vi "QWTB Algorithms Filter Set Config.vi"(9 "new algorithm config section data":string, 10 "algorithm name":string, 11 "info data":string) -> (3 "info data out":string)   [LabVIEW 2020]
uses:
  octave/infolib/infolib.lvlib
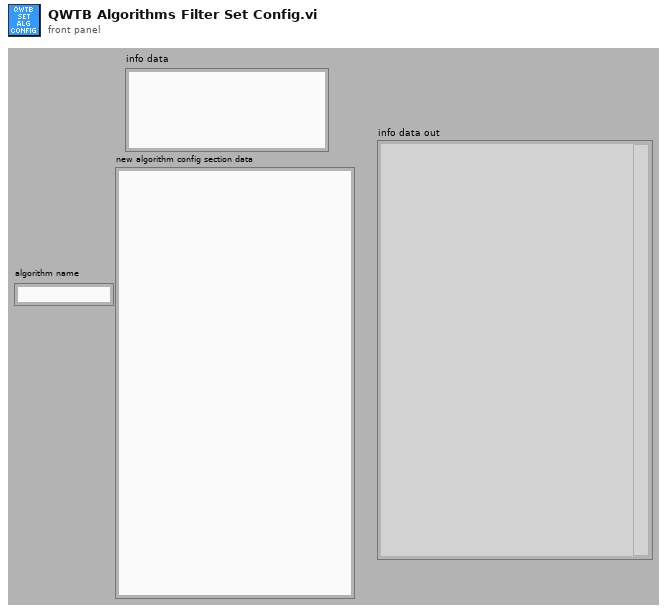
[diagram p1: front panel]
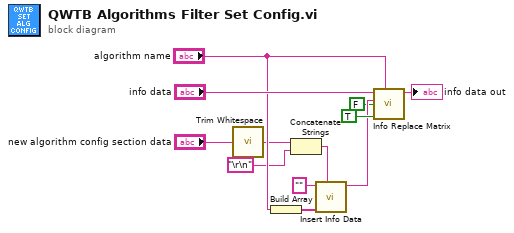
[diagram p0: block diagram]
diagram:
  n1 = call <vilib>:"Trim Whitespace.vi"("string"="new algorithm config section data") -> ("trimmed string"=w3:string)  [unwired: 1 in]
  n2 = Build Array("algorithm name") -> (w8:string[])
  n3 = Concatenate Strings(w3, "\r\n") -> (w2:string)
  n4 = call "Insert Info Data.vi"("info data to insert"=w2, "sections"=w8, "info data"="") -> ("info data out"=w7:string)  [unwired: 7 in, 1 out]
  n5 = call "Info Replace Matrix.vi"("key description to replace"="algorithm name", "Is Section (False)"=TRUE, "Allow indent (True)"=FALSE, "info data to paste"=w7, "info data in"="info data") -> ("info data out"=→"info data out":string)  [unwired: 6 in]
